vi "postgres_date_to_timestamp.vi"(8 "error in (no error)":errorcluster, 10 "utc":bool, 11 "postgres_date":string) -> (0 "error out":errorcluster, 3 "date_time":dbl format="%^<%H:%M:%S%4u %m/%d/%y>T")   [LabVIEW 2015, in "lv-example-postgres.lvlib"]
uses:
  lv-example-postgres.lvlib
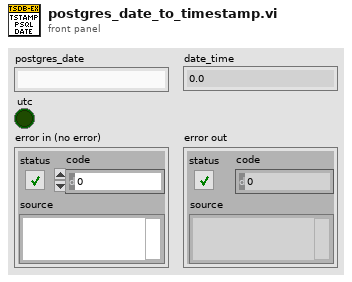
[diagram p1: front panel]
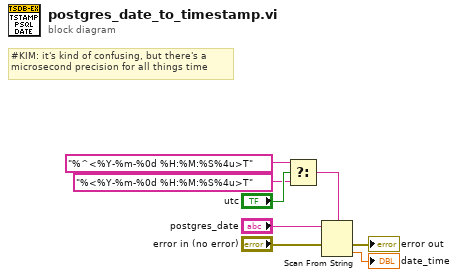
[diagram p0: block diagram]
diagram:
  # "#KIM: it's kind of confusing, but there's a \nmicrosecond precision for all things time"
  n1 = Select(t="%^<%Y-%m-%0d %H:%M:%S%4u>T", s="utc", f="%<%Y-%m-%0d %H:%M:%S%4u>T") -> (s? t:f=w3:string)
  n2 = Scan From String(format string=w3, input string="postgres_date", error in="error in (no error)") -> (error out=→"error out":errorcluster, output 1=→"date_time":dbl)  [unwired: 2 in, 2 out]
